vi "Idle_ParseStringCommand.vi"(3 "error in":errorcluster, 5 "Input Command":string="Command_Remainder") -> (0 "error out":errorcluster, 1 "Command":string="Command", 2 "Remaining String":string="Remainder")   [LabVIEW 2012]
uses:
  <vilib>/regexp/Match Regular Expression.xnode
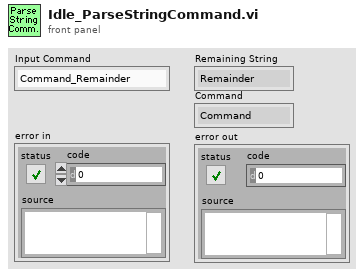
[diagram p1: front panel]
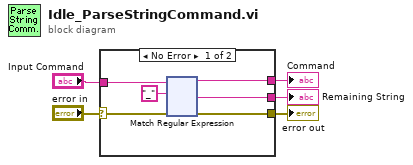
[diagram p0: block diagram]
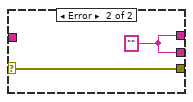
[diagram p2: hidden frame]
diagram:
  n1 = case shown="No Error" "error in" {
    selector: "error in" -> [w10 w123]
    tunnel: "Input Command" -> [w11 _]
    tunnel: [w8 w124] -> w1
    tunnel: [w7 w124] -> w2
    tunnel: [w6 w123] -> w3
    frame No Error {
      n2 = xnode "Match Regular Expression"("input string"=w11, "regular expression"="_", "error in"=w10) -> ("before match"=w8:string, "after match"=w7:string, "error out"=w6:errorcluster)  [unwired: 3 in, 2 out]
    }
    frame Error {
      w124 = ""
    }
  }
  "error out" <- w3
  "Remaining String" <- w2
  "Command" <- w1
